vi "SENS_MIX_LOAD.vi"(0 "VISA IN":refnum<visa-resource-name>, 5 "error in":errorcluster, 7 "Channel":i32, 11 "FileName":string) -> (14 "VISA Out":refnum<visa-resource-name>, 19 "error out":errorcluster)   [LabVIEW 2018, in "PNA-X.lvlib"]
doc: "SENSe:PATH:CONFiguration:DELete <string>\n(Write-only) Deletes the specified configuration name from the PNA. The factory configurations cannot be deleted. This is the only method of distinguishing a factory configuration from a user-named configuration.\n \nParameters\n \n \n<string>\n Configuration name to be deleted.\n \nExamples\n SENS:PATH:CONF:DEL \"MyMixer\"\n \nReturn Type\n Not Applicable\n \nDefault\n Not Applicable"
uses:
  PNA-X.lvlib
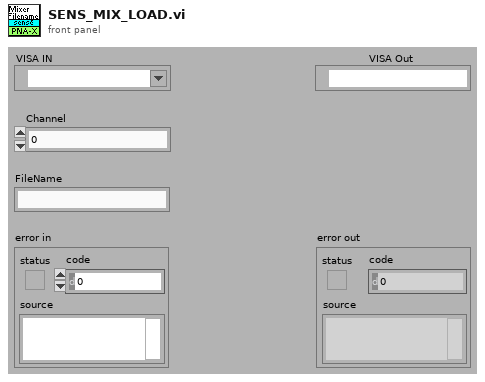
[diagram p1: front panel]
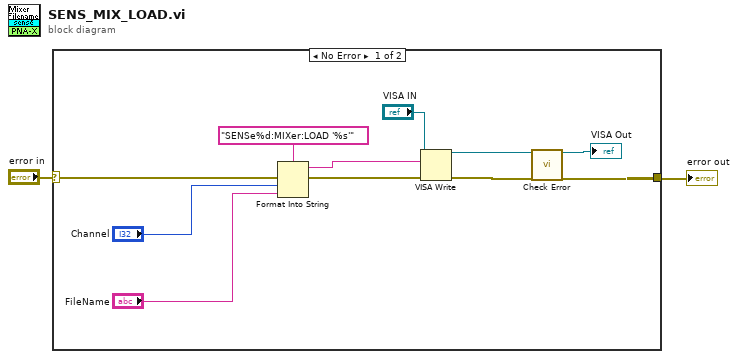
[diagram p0: block diagram]
diagram:
  n1 = case shown="No Error" "error in" {
    selector: "error in" -> [w11 w14]
    tunnel: [w5 w14] -> w1
    frame No Error {
      n2 = Format Into String(format string="SENSe%d:MIXer:LOAD '%s'" ("Cmdline"), error in=w11, "Channel", "FileName") -> (resulting string=w10:string, error out=w12:errorcluster)  [unwired: 1 in]
      n3 = VISA Write(VISA resource name="VISA IN", write buffer=w10, error in (no error)=w12) -> (VISA resource name out=w3:refnum<visa-resource-name>, error out=w6:errorcluster)  [unwired: 1 out]
      n4 = call "Check Error.vi"("VISA Resource Name"=w3, "error in (no error)"=w6) -> ("dup VISA session"=→"VISA Out":refnum<visa-resource-name>, "error out"=w5:errorcluster)  [unwired: 16 in]
    }
    frame Error {
    }
  }
  "error out" <- w1
